vi "write_zssp.vi"() -> (0 "sortie d'erreur":errorcluster)   [LabVIEW 2011]
panel:
  out "pdir_path":path
  in  "Chemin":path
  out "power value":dbl
  out "shutter 2":bool
  out "shutter 1":bool
  out "z value":dbl
  out "chanel num":u8
  out "position num":u8
  in  "power":dbl
  in  "shutter2":bool
  in  "shutter1":bool
  in  "z":dbl
  in  "chanelnum":u8
  in  "posnum":u8
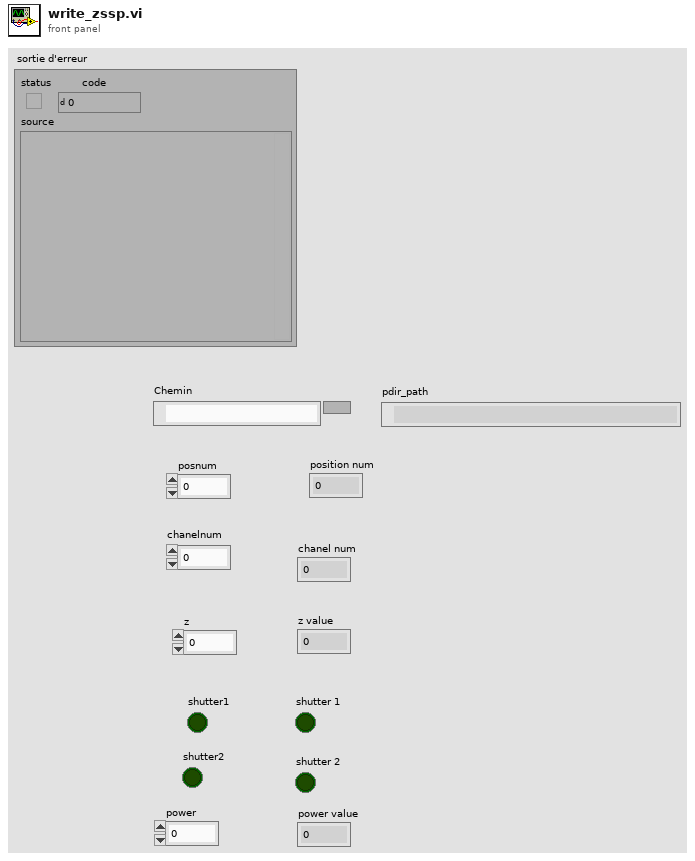
[diagram p1: front panel]
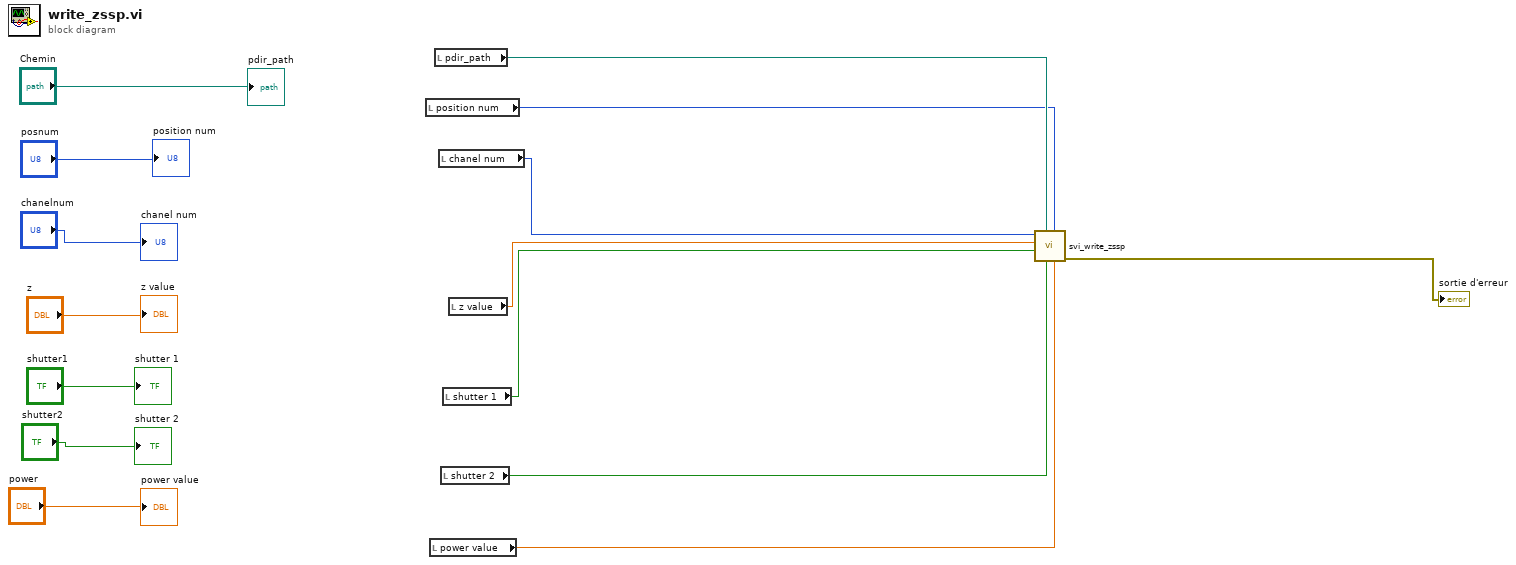
[diagram p0: block diagram]
diagram:
  n1 = local read "position num"() -> (w3:u8)
  n2 = local read "power value"() -> (w5:dbl)
  n3 = local read "pdir_path"() -> (w4:path)
  n4 = local read "chanel num"() -> (w2:u8)
  n5 = local read "shutter 2"() -> (w6:bool)
  n6 = local read "shutter 1"() -> (w7:bool)
  n7 = local read "z value"() -> (w8:dbl)
  n8 = call "svi_write_zssp.vi"("power value"=w5, "position num"=w3, "shutter en entrée"=w6, "pdir_path"=w4, "shutter 1"=w7, "z value"=w8, "chanel num"=w2) -> ("sortie d'erreur"=→"sortie d'erreur":errorcluster)  [unwired: 4 in]
  "position num" <- "posnum"
  "chanel num" <- "chanelnum"
  "z value" <- "z"
  "shutter 1" <- "shutter1"
  "shutter 2" <- "shutter2"
  "power value" <- "power"
  "pdir_path" <- "Chemin"
